vi "Test Matching String Test.vi"(8 "error in (no error)":errorcluster, 11 "LUnit Test Case V2 Test Double In":refnum<class "Test Case Test Double.lvclass">) -> (0 "error out":errorcluster, 3 "LUnit Test Case V2 Test Double Out":refnum<class "Test Case Test Double.lvclass">)   [LabVIEW 2020, in "Test Case Test Double.lvclass"]
uses:
  Test Case Test Double.lvclass
  Test Case Test Double.lvclass/Test Case Test Double.ctl
  source/Core/Advanced Assertions/Advanced Assertions.lvlib
  C:/git/astemes-lunit/source/LUnit Test Case.lvclass
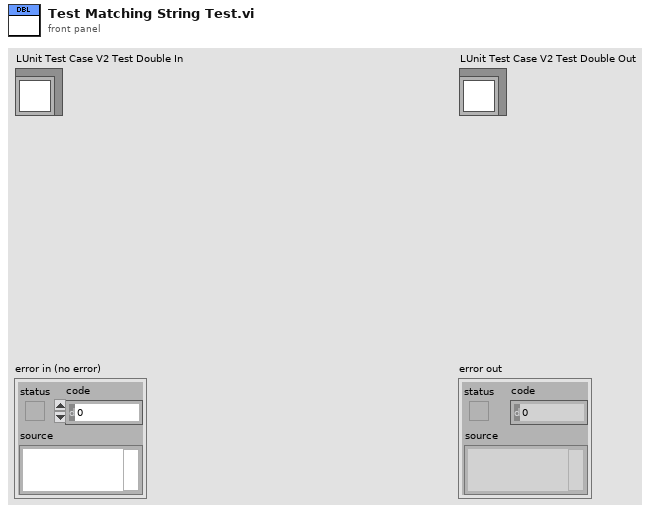
[diagram p1: front panel]
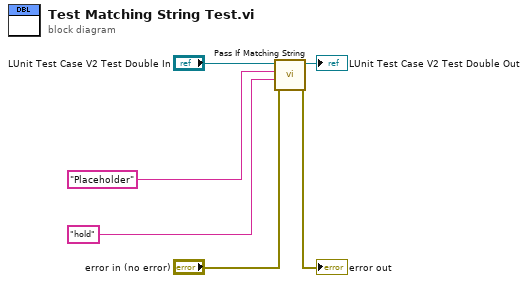
[diagram p0: block diagram]
diagram:
  n1 = call "Pass If Matching String.vi"("error in (no error)"="error in (no error)", "Regular Expression"="hold", "String"="Placeholder", "LUnit Test Case In"="LUnit Test Case V2 Test Double In") -> ("error out"=→"error out":errorcluster, "LUnit Test Case Out"=→"LUnit Test Case V2 Test Double Out":refnum<class "Test Case Test Double.lvclass">)  [unwired: 6 in]
